vi "IMAQ ReadFile 2.vi"(6 "Use File Path Image Type":bool=TRUE, 7 "File Path":path, 8 "error in (no error)":errorcluster, 9 "File Options":T1 {"Optional Max Value" format="%.2f"; "Optional Min Value" format="%.2f"; "File Data Type" items=["1 bit", "2 bits", "4 bits", "8 bits", "16 bits (unsigned)", "16 bits (signed)", "16 bits (RGB chunky)", "24 bits (RGB chunky)", "24 bits (RGB planar)", "32 bits (unsigned)", "32 bits (signed)", "32 bits (RGB chunky)", "32 bits (float)", "48 bits (Complex 2x24 int)", "64 bits (Complex 2x32 float)", "32 bits (HSL)"]; "Read Raw File" items=["Don't Read Raw File ", "Read Raw File"]}, 10 "Load Color Palette? (No)":bool, 11 "Image":T2) -> (0 "error out":errorcluster, 1 "File Data Type out":i32, 2 "File Type out":string, 3 "Image Out":T2, 5 "Color Palette out":cluster{"Red":u8, "Green":u8, "Blue":u8}[](array[cluster]))   [LabVIEW 2019]
doc: "Reads an image file. The file format can be a standard format (BMP, TIFF, JPEG, JPEG2000, PNG, and AIPD) or a nonstandard format known to the user."
uses:
  <vilib>/vision/Image Controls.llb/IMAQ Image.ctl
  nivision.dll
panel:
  # "- Yes\n- No"
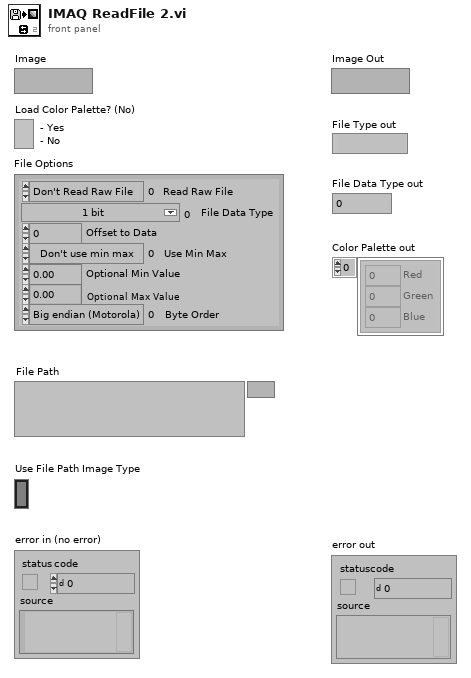
[diagram p1: front panel]
types:
  T1 = cluster{"Read Raw File":i32, "File Data Type":u32, "Offset to Data":i32, "Use Min Max":enum32{"Don't use min max", "Use file values", "Use optional values"}, "Optional Min Value":sgl, "Optional Max Value":sgl, "Byte Order":enum32{"Big endian (Motorola)", "Little endian (Intel)"}}
  T2 = typedef "IMAQ Image.ctl" = refnum<image>
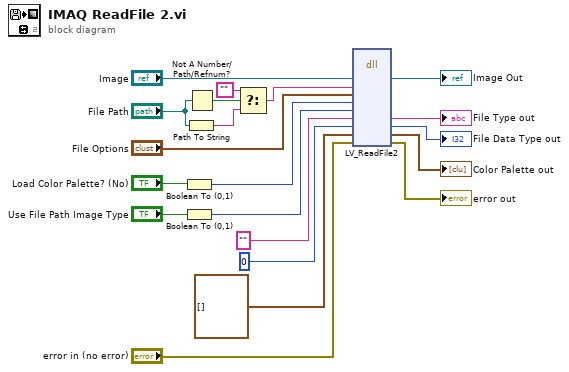
[diagram p0: block diagram]
diagram:
  n1 = Boolean To (0,1)(Boolean="Load Color Palette? (No)") -> (0, 1=w17:i16)
  n2 = Boolean To (0,1)(Boolean="Use File Path Image Type") -> (0, 1=w1:i16)
  n3 = Path To String(path="File Path") -> (string=w7:string)
  n4 = Not A Number/Path/Refnum?(number/path/refnum="File Path") -> (NaN/Path/Refnum?=w6:bool)
  n5 = Select(t="", s=w6, f=w7) -> (s? t:f=w4:string)
  n6 = dll-call lib="nivision.*" fn="LV_ReadFile2"("Image"="Image", "Filepath"=w4, "FileOptions"="File Options", "LoadColorPalette"=w17, "_fileTypeSrc"=w1, "FileType"="" ("File Type"), "FileDataType"=0 ("File Data Type"), "ColorPalette"=cluster{"Red":u8, "Green":u8, "Blue":u8}[] [] ("Color Palette"), "error"="error in (no error)") -> ("Image"=→"Image Out":T2, "FileType"=→"File Type out":string, "FileDataType"=→"File Data Type out":i32, "ColorPalette"=→"Color Palette out":cluster{"Red":u8, "Green":u8, "Blue":u8}[], "error"=→"error out":errorcluster)  [unwired: 7 in, 3 out]
